vi "总磷氨氮测量数据储存.vi"   [LabVIEW 2016, in "氨氮.lvlib"]
types:
  T1 = enum16{"维护数据", "水样测试", "标样核查", "零点核查", "跨度核查", "空白测试", "平行样测试", "加标回收", "空白校准", "标样校准", "初始化（清洗）"}
  T2 = cluster{"时间标识":timestamp, "监测值":sgl, "单位":u16, "数据标识":string, "因子编码":u32, "标样参考值":sgl, "F0":sgl, "F1":sgl, "F2":sgl, "F3":sgl, "温度":sgl, "湿度":sgl, "量程标识":string}
  T3 = cluster{"运行模式":enum16{"维护模式", "常规模式", "应急模式", "质控模式"}}
  T4 = cluster{"系统时间":timestamp, "工作状态":enum16{"空闲", "水样测试", "标样核查", "零点核查", "跨度核查", "空白测试", "平行样测试", "加标回收", "空白校准", "标样校准", "初始化（清洗）"}, "测量模式":enum16{"待机", "连续模式", "周期模式", "定点模式", "受控模式", "手动模式"}, "告警代码":enum16{"无告警", "缺试剂告警", "缺水样告警", "缺蒸馏水告警", "缺标液告警", "仪表漏液告警", "标定异常告警", "超量程告警", "加热异常", "低试剂预警", "超上限告警", "超下限告警", "仪表内部其他异常", "滴定异常告警", "电极异常告警", "量程切换告警", "参数设置告警", "PH电极电位异常", "电导率电极异常", "浊度光度异常", "溶解氧电极异常", "溶解氧光强异常", "温度异常告警", "PH异常告警", "溶解氧异常告警", "电导率异常告警", "浊度异常告警", "叶绿素异常告警", "藻密度异常告警", "蓝绿藻异常告警", "ORP异常告警", "氨氮异常告警", "清洁刷异常告警", "SD卡异常告警", "蓝牙异常告警", "Wifi异常告警", "流程异常告警"}, "故障代码":enum16{"无故障", "电机故障", "温度故障", "通讯故障", "滴定故障"}, "日志代码":u16, "软件版本":u16, "F0":sgl, "F1":sgl, "F2":sgl, "F3":sgl, "T":sgl, "H":sgl, "id":u16, "flowid":u16, "量程":u16, "总磷控温温度1":sgl, "营养盐控温温度2":sgl, "ADC":sgl}
  T5 = enum16{"空闲", "水样测试", "标样核查", "零点核查", "跨度核查", "空白测试", "平行样测试", "加标回收", "空白校准", "标样校准", "初始化（清洗）"}
  T6 = cluster{"因子编码":u32, "单位":u16, "标样参考值":sgl, "水样数据时间":timestamp, "水样实测值":sgl, "水样数据标识":string, "标样数据时间":timestamp, "标样实测值":sgl, "标样数据标识":string, "空白数据时间":timestamp, "空白实测值":sgl, "空白数据标识":string, "零点核查数据时间":timestamp, "零点核查实测值":sgl, "零点核查数据标识":string, "跨度核查数据时间":timestamp, "跨度核查实测值":sgl, "跨度核查数据标识":string, "加标回收数据时间":timestamp, "加标回收实测值":sgl, "加标回收数据标识":string, "平行样数据时间":timestamp, "平行样实测值":sgl, "平行样数据标识":string}
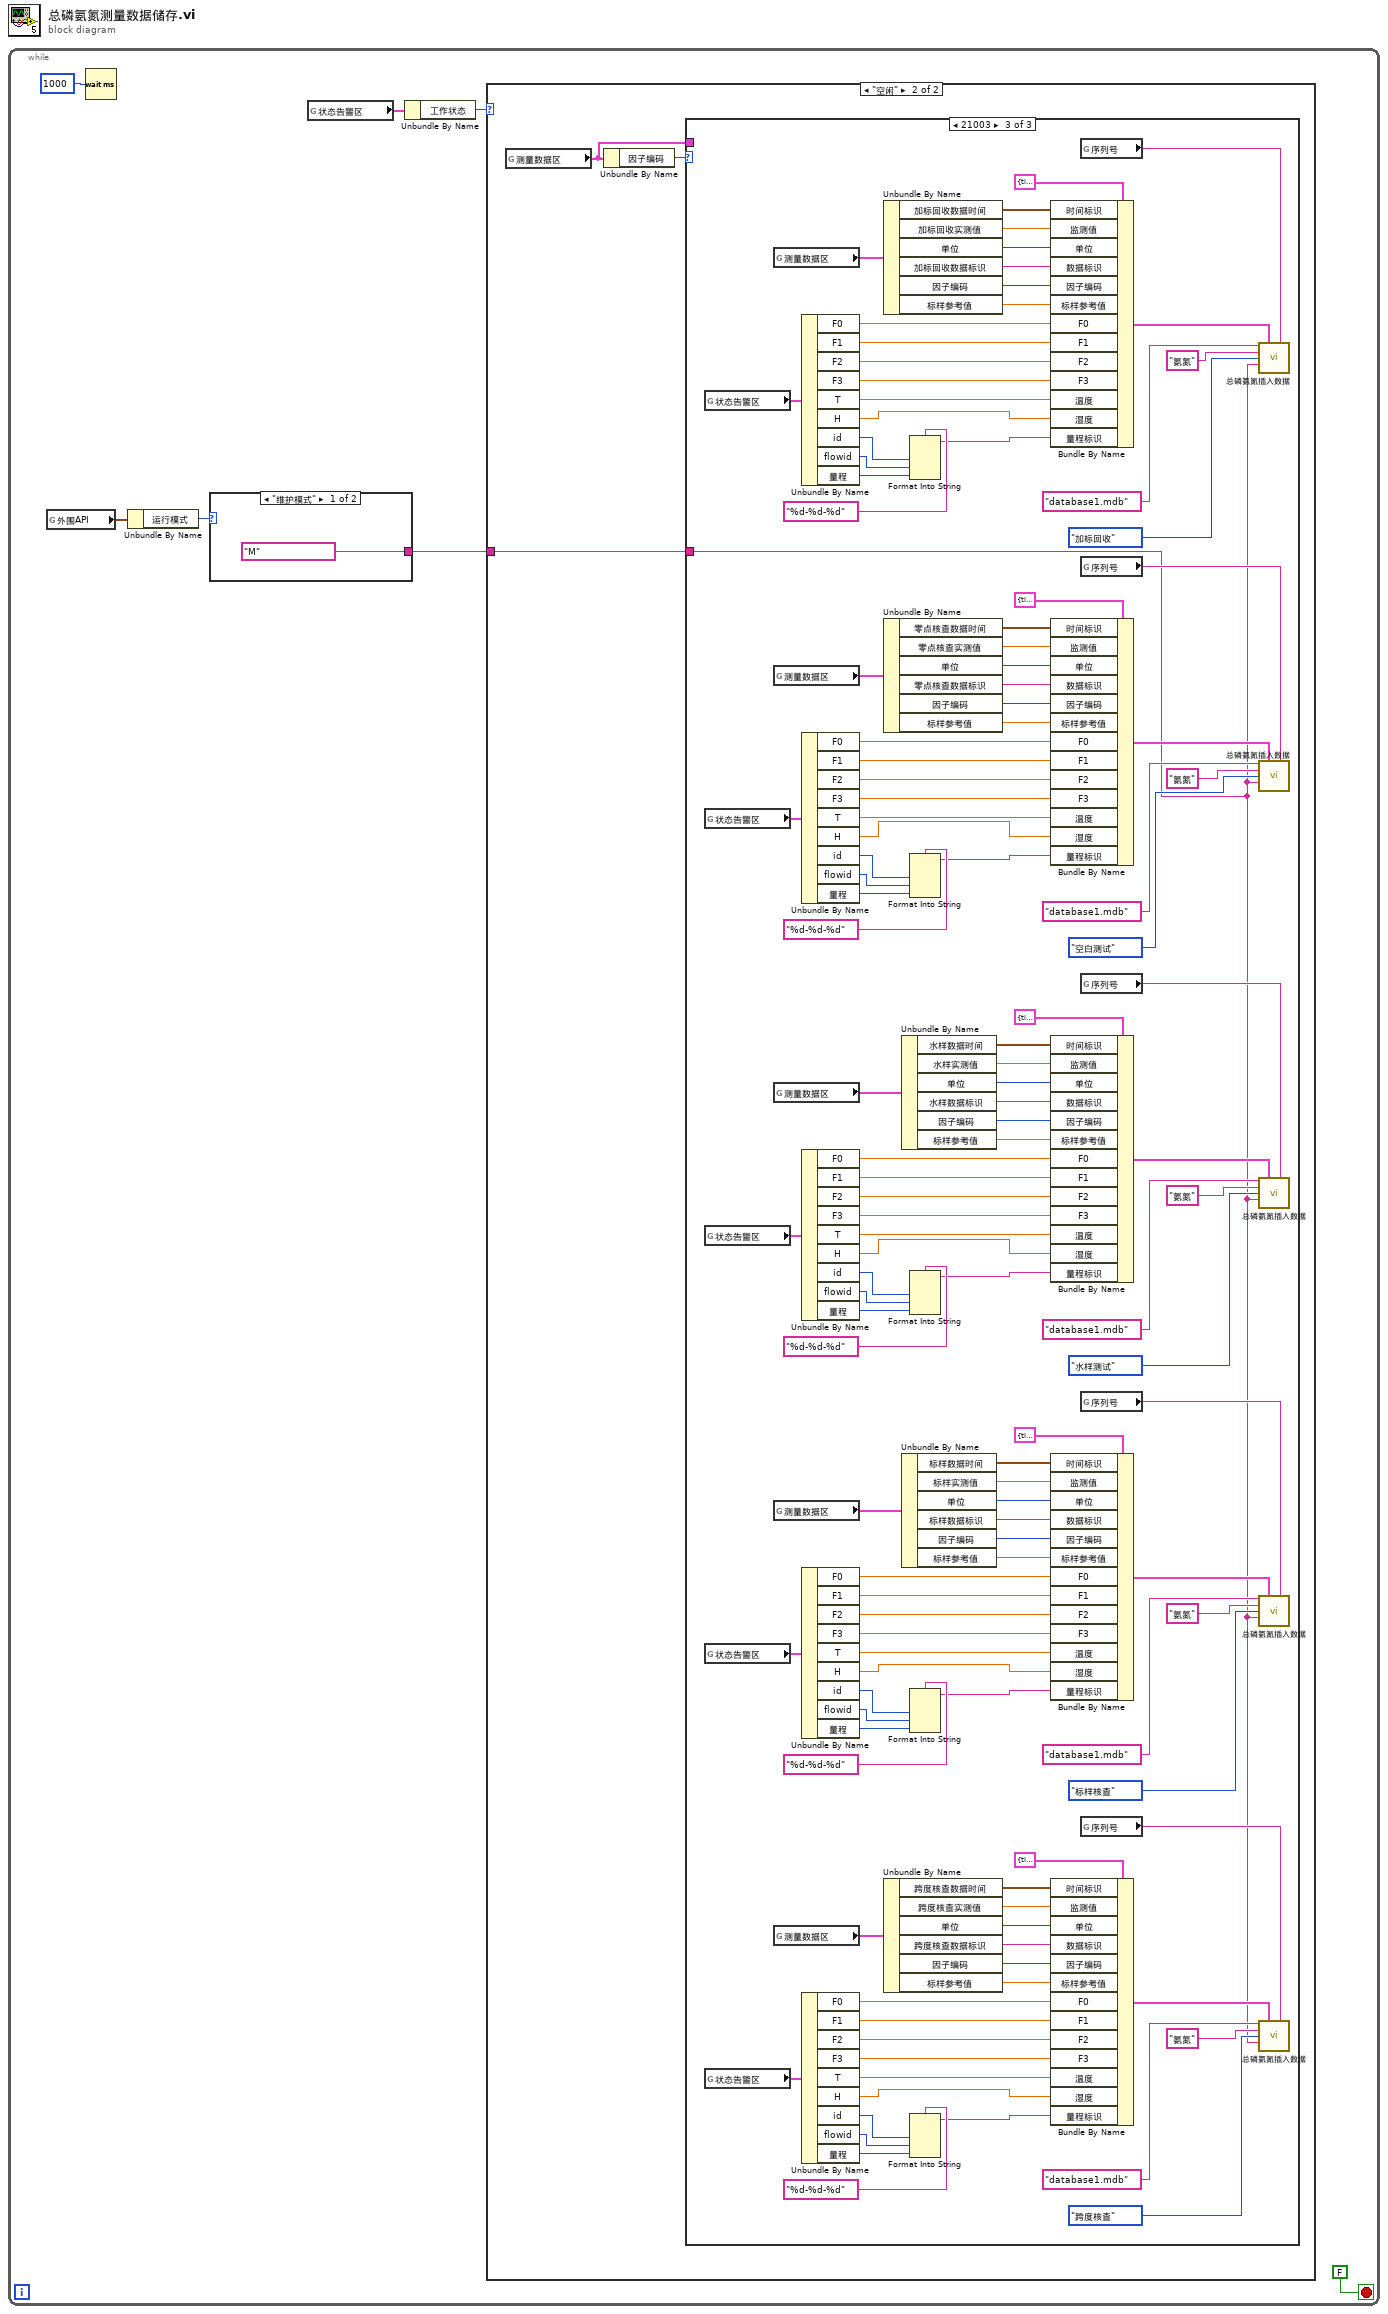
[diagram p0: block diagram]
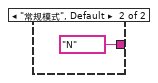
[diagram p2: hidden frame]
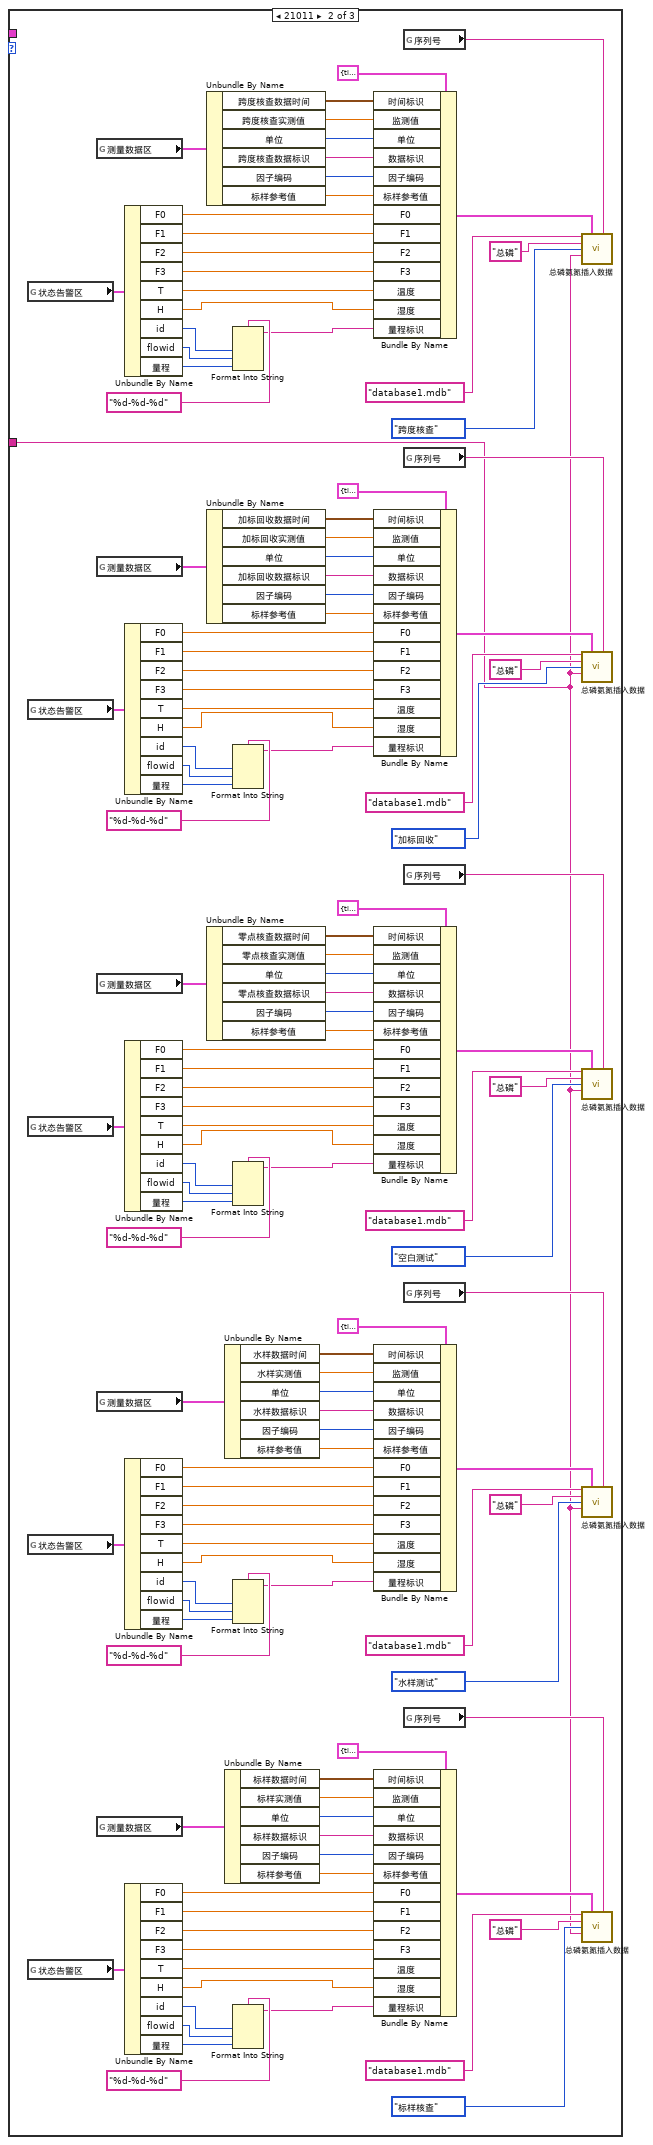
[diagram p5: hidden frame]
diagram:
  n1 = while {
    stop <- FALSE stop-if-true
    n2 = global read "VAR氨氮全局变量.vi" "外围API"() -> (w2:T3)
    n3 = Wait (ms)(milliseconds to wait=u32 1000 ("等待时间（毫秒）")) -> ()  [unwired: 1 out]
    n4 = Unbundle By Name(w2) -> ("运行模式"=w1:enum16{"维护模式", "常规模式", "应急模式", "质控模式"})
    n5 = case shown="\"维护模式\"" w1 {
      tunnel: ["M" ("数据标记表") "N" ("数据标记表")] -> w3
      frame "维护模式" {
      }
      frame "常规模式", Default {
      }
    }
    n6 = global read "VAR氨氮全局变量.vi" "状态告警区"() -> (w5:T4)
    n7 = Unbundle By Name(w5) -> ("工作状态"=w4:T5)
    n8 = case shown="\"空闲\"" w4 {
      tunnel: w3 -> [_ w10]
      frame Default {
      }
      frame "空闲" {
        n9 = global read "VAR氨氮全局变量.vi" "测量数据区"() -> (w12:T6)
        n10 = Unbundle By Name(w12) -> ("因子编码"=w11:u32)
        n11 = case shown="21003" w11 {
          tunnel: w12 -> [_ _ _]
          tunnel: w10 -> [_ w13 w139]
          frame Default {
          }
          frame 21011 {
            n12 = global read "VAR氨氮全局变量.vi" "状态告警区"() -> (w77:T4)
            n13 = global read "VAR氨氮全局变量.vi" "状态告警区"() -> (w59:T4)
            n14 = global read "VAR氨氮全局变量.vi" "状态告警区"() -> (w92:T4)
            n15 = global read "VAR氨氮全局变量.vi" "状态告警区"() -> (w131:T4)
            n16 = global read "VAR氨氮全局变量.vi" "状态告警区"() -> (w110:T4)
            n17 = global read "VAR氨氮全局变量.vi" "测量数据区"() -> (w84:T6)
            n18 = global read "VAR氨氮全局变量.vi" "测量数据区"() -> (w66:T6)
            n19 = global read "VAR氨氮全局变量.vi" "测量数据区"() -> (w85:T6)
            n20 = global read "VAR氨氮全局变量.vi" "测量数据区"() -> (w138:T6)
            n21 = global read "VAR氨氮全局变量.vi" "测量数据区"() -> (w103:T6)
            n22 = Unbundle By Name(w77) -> ("F0"=w76:sgl, "F1"=w75:sgl, "F2"=w74:sgl, "F3"=w73:sgl, "T"=w72:sgl, "H"=w71:sgl, "id"=w40:u16, "flowid"=w39:u16, "量程"=w38:u16)
            n23 = Unbundle By Name(w59) -> ("F0"=w58:sgl, "F1"=w57:sgl, "F2"=w56:sgl, "F3"=w55:sgl, "T"=w54:sgl, "H"=w53:sgl, "id"=w46:u16, "flowid"=w45:u16, "量程"=w44:u16)
            n24 = Unbundle By Name(w92) -> ("F0"=w93:sgl, "F1"=w94:sgl, "F2"=w95:sgl, "F3"=w96:sgl, "T"=w97:sgl, "H"=w98:sgl, "id"=w33:u16, "flowid"=w34:u16, "量程"=w35:u16)
            n25 = Unbundle By Name(w131) -> ("F0"=w130:sgl, "F1"=w129:sgl, "F2"=w128:sgl, "F3"=w127:sgl, "T"=w126:sgl, "H"=w125:sgl, "id"=w20:u16, "flowid"=w21:u16, "量程"=w22:u16)
            n26 = Unbundle By Name(w110) -> ("F0"=w111:sgl, "F1"=w112:sgl, "F2"=w113:sgl, "F3"=w114:sgl, "T"=w115:sgl, "H"=w116:sgl, "id"=w28:u16, "flowid"=w27:u16, "量程"=w26:u16)
            n27 = Unbundle By Name(w84) -> ("跨度核查数据时间"=w83:timestamp, "跨度核查实测值"=w82:sgl, "单位"=w81:u16, "跨度核查数据标识"=w80:string, "因子编码"=w79:u32, "标样参考值"=w78:sgl)
            n28 = Unbundle By Name(w66) -> ("加标回收数据时间"=w65:timestamp, "加标回收实测值"=w64:sgl, "单位"=w63:u16, "加标回收数据标识"=w62:string, "因子编码"=w61:u32, "标样参考值"=w60:sgl)
            n29 = Unbundle By Name(w85) -> ("零点核查数据时间"=w86:timestamp, "零点核查实测值"=w87:sgl, "单位"=w88:u16, "零点核查数据标识"=w89:string, "因子编码"=w90:u32, "标样参考值"=w91:sgl)
            n30 = Unbundle By Name(w138) -> ("水样数据时间"=w137:timestamp, "水样实测值"=w136:sgl, "单位"=w135:u16, "水样数据标识"=w134:string, "因子编码"=w133:u32, "标样参考值"=w132:sgl)
            n31 = Unbundle By Name(w103) -> ("标样数据时间"=w104:timestamp, "标样实测值"=w105:sgl, "单位"=w106:u16, "标样数据标识"=w107:string, "因子编码"=w108:u32, "标样参考值"=w109:sgl)
            n32 = Format Into String(format string="%d-%d-%d" ("格式字符串"), w40, w39, w38) -> (resulting string=w37:string)  [unwired: 2 in, 1 out]
            n33 = Format Into String(format string="%d-%d-%d" ("格式字符串"), w46, w45, w44) -> (resulting string=w43:string)  [unwired: 2 in, 1 out]
            n34 = Format Into String(format string="%d-%d-%d" ("格式字符串"), w33, w34, w35) -> (resulting string=w31:string)  [unwired: 2 in, 1 out]
            n35 = Format Into String(format string="%d-%d-%d" ("格式字符串"), w20, w21, w22) -> (resulting string=w19:string)  [unwired: 2 in, 1 out]
            n36 = Format Into String(format string="%d-%d-%d" ("格式字符串"), w28, w27, w26) -> (resulting string=w25:string)  [unwired: 2 in, 1 out]
            n37 = Bundle By Name(cluster=T2 {"时间标识"=timestamp(0 s since 1904-01-01), "监测值"=0.0, "单位"=0, "数据标识"="", "因子编码"=0, "标样参考值"=0.0, "F0"=0.0, "F1"=0.0, "F2"=0.0, "F3"=0.0, "温度"=0.0, "湿度"=0.0, "量程标识"=""} ("data"), "时间标识"=w83, "监测值"=w82, "单位"=w81, "数据标识"=w80, "因子编码"=w79, "标样参考值"=w78, "F0"=w76, "F1"=w75, "F2"=w74, "F3"=w73, "温度"=w72, "湿度"=w71, "量程标识"=w37) -> (w70:T2)
            n38 = Bundle By Name(cluster=T2 {"时间标识"=timestamp(0 s since 1904-01-01), "监测值"=0.0, "单位"=0, "数据标识"="", "因子编码"=0, "标样参考值"=0.0, "F0"=0.0, "F1"=0.0, "F2"=0.0, "F3"=0.0, "温度"=0.0, "湿度"=0.0, "量程标识"=""} ("data"), "时间标识"=w65, "监测值"=w64, "单位"=w63, "数据标识"=w62, "因子编码"=w61, "标样参考值"=w60, "F0"=w58, "F1"=w57, "F2"=w56, "F3"=w55, "温度"=w54, "湿度"=w53, "量程标识"=w43) -> (w52:T2)
            n39 = Bundle By Name(cluster=T2 {"时间标识"=timestamp(0 s since 1904-01-01), "监测值"=0.0, "单位"=0, "数据标识"="", "因子编码"=0, "标样参考值"=0.0, "F0"=0.0, "F1"=0.0, "F2"=0.0, "F3"=0.0, "温度"=0.0, "湿度"=0.0, "量程标识"=""} ("data"), "时间标识"=w86, "监测值"=w87, "单位"=w88, "数据标识"=w89, "因子编码"=w90, "标样参考值"=w91, "F0"=w93, "F1"=w94, "F2"=w95, "F3"=w96, "温度"=w97, "湿度"=w98, "量程标识"=w31) -> (w99:T2)
            n40 = Bundle By Name(cluster=T2 {"时间标识"=timestamp(0 s since 1904-01-01), "监测值"=0.0, "单位"=0, "数据标识"="", "因子编码"=0, "标样参考值"=0.0, "F0"=0.0, "F1"=0.0, "F2"=0.0, "F3"=0.0, "温度"=0.0, "湿度"=0.0, "量程标识"=""} ("data"), "时间标识"=w137, "监测值"=w136, "单位"=w135, "数据标识"=w134, "因子编码"=w133, "标样参考值"=w132, "F0"=w130, "F1"=w129, "F2"=w128, "F3"=w127, "温度"=w126, "湿度"=w125, "量程标识"=w19) -> (w124:T2)
            n41 = Bundle By Name(cluster=T2 {"时间标识"=timestamp(0 s since 1904-01-01), "监测值"=0.0, "单位"=0, "数据标识"="", "因子编码"=0, "标样参考值"=0.0, "F0"=0.0, "F1"=0.0, "F2"=0.0, "F3"=0.0, "温度"=0.0, "湿度"=0.0, "量程标识"=""} ("data"), "时间标识"=w104, "监测值"=w105, "单位"=w106, "数据标识"=w107, "因子编码"=w108, "标样参考值"=w109, "F0"=w111, "F1"=w112, "F2"=w113, "F3"=w114, "温度"=w115, "湿度"=w116, "量程标识"=w25) -> (w117:T2)
            n42 = global read "VAR氨氮全局变量.vi" "序列号"() -> (w15:string)
            n43 = global read "VAR氨氮全局变量.vi" "序列号"() -> (w14:string)
            n44 = global read "VAR氨氮全局变量.vi" "序列号"() -> (w16:string)
            n45 = global read "VAR氨氮全局变量.vi" "序列号"() -> (w18:string)
            n46 = global read "VAR氨氮全局变量.vi" "序列号"() -> (w17:string)
            n47 = call "总磷氨氮插入数据.vi"("database"="database1.mdb", "data"=w70, "SN"=w15, "table"="总磷", "测量模式"=T1."跨度核查", "数据标记表"=w13) -> ()  [unwired: 9 in, 1 out]
            n48 = call "总磷氨氮插入数据.vi"("database"="database1.mdb", "data"=w52, "SN"=w14, "table"="总磷", "测量模式"=T1."加标回收", "数据标记表"=w13) -> ()  [unwired: 9 in, 1 out]
            n49 = call "总磷氨氮插入数据.vi"("database"="database1.mdb", "data"=w99, "SN"=w16, "table"="总磷", "测量模式"=T1."空白测试", "数据标记表"=w13) -> ()  [unwired: 9 in, 1 out]
            n50 = call "总磷氨氮插入数据.vi"("database"="database1.mdb", "data"=w124, "SN"=w18, "table"="总磷", "测量模式"=T1."水样测试", "数据标记表"=w13) -> ()  [unwired: 9 in, 1 out]
            n51 = call "总磷氨氮插入数据.vi"("database"="database1.mdb", "data"=w117, "SN"=w17, "table"="总磷", "测量模式"=T1."标样核查", "数据标记表"=w13) -> ()  [unwired: 9 in, 1 out]
          }
          frame 21003 {
            n52 = global read "VAR氨氮全局变量.vi" "状态告警区"() -> (w185:T4)
            n53 = global read "VAR氨氮全局变量.vi" "状态告警区"() -> (w218:T4)
            n54 = global read "VAR氨氮全局变量.vi" "状态告警区"() -> (w257:T4)
            n55 = global read "VAR氨氮全局变量.vi" "状态告警区"() -> (w236:T4)
            n56 = global read "VAR氨氮全局变量.vi" "状态告警区"() -> (w203:T4)
            n57 = global read "VAR氨氮全局变量.vi" "测量数据区"() -> (w192:T6)
            n58 = global read "VAR氨氮全局变量.vi" "测量数据区"() -> (w211:T6)
            n59 = global read "VAR氨氮全局变量.vi" "测量数据区"() -> (w264:T6)
            n60 = global read "VAR氨氮全局变量.vi" "测量数据区"() -> (w229:T6)
            n61 = global read "VAR氨氮全局变量.vi" "测量数据区"() -> (w210:T6)
            n62 = Unbundle By Name(w185) -> ("F0"=w184:sgl, "F1"=w183:sgl, "F2"=w182:sgl, "F3"=w181:sgl, "T"=w180:sgl, "H"=w179:sgl, "id"=w160:u16, "flowid"=w159:u16, "量程"=w158:u16)
            n63 = Unbundle By Name(w218) -> ("F0"=w219:sgl, "F1"=w220:sgl, "F2"=w221:sgl, "F3"=w222:sgl, "T"=w223:sgl, "H"=w224:sgl, "id"=w148:u16, "flowid"=w147:u16, "量程"=w146:u16)
            n64 = Unbundle By Name(w257) -> ("F0"=w256:sgl, "F1"=w255:sgl, "F2"=w254:sgl, "F3"=w253:sgl, "T"=w252:sgl, "H"=w251:sgl, "id"=w173:u16, "flowid"=w172:u16, "量程"=w171:u16)
            n65 = Unbundle By Name(w236) -> ("F0"=w237:sgl, "F1"=w238:sgl, "F2"=w239:sgl, "F3"=w240:sgl, "T"=w241:sgl, "H"=w242:sgl, "id"=w166:u16, "flowid"=w165:u16, "量程"=w164:u16)
            n66 = Unbundle By Name(w203) -> ("F0"=w202:sgl, "F1"=w201:sgl, "F2"=w200:sgl, "F3"=w199:sgl, "T"=w198:sgl, "H"=w197:sgl, "id"=w154:u16, "flowid"=w153:u16, "量程"=w152:u16)
            n67 = Unbundle By Name(w192) -> ("加标回收数据时间"=w191:timestamp, "加标回收实测值"=w190:sgl, "单位"=w189:u16, "加标回收数据标识"=w188:string, "因子编码"=w187:u32, "标样参考值"=w186:sgl)
            n68 = Unbundle By Name(w211) -> ("零点核查数据时间"=w212:timestamp, "零点核查实测值"=w213:sgl, "单位"=w214:u16, "零点核查数据标识"=w215:string, "因子编码"=w216:u32, "标样参考值"=w217:sgl)
            n69 = Unbundle By Name(w210) -> ("跨度核查数据时间"=w209:timestamp, "跨度核查实测值"=w208:sgl, "单位"=w207:u16, "跨度核查数据标识"=w206:string, "因子编码"=w205:u32, "标样参考值"=w204:sgl)
            n70 = Unbundle By Name(w264) -> ("水样数据时间"=w263:timestamp, "水样实测值"=w262:sgl, "单位"=w261:u16, "水样数据标识"=w260:string, "因子编码"=w259:u32, "标样参考值"=w258:sgl)
            n71 = Unbundle By Name(w229) -> ("标样数据时间"=w230:timestamp, "标样实测值"=w231:sgl, "单位"=w232:u16, "标样数据标识"=w233:string, "因子编码"=w234:u32, "标样参考值"=w235:sgl)
            n72 = Format Into String(format string="%d-%d-%d" ("格式字符串"), w160, w159, w158) -> (resulting string=w157:string)  [unwired: 2 in, 1 out]
            n73 = Format Into String(format string="%d-%d-%d" ("格式字符串"), w148, w147, w146) -> (resulting string=w145:string)  [unwired: 2 in, 1 out]
            n74 = Format Into String(format string="%d-%d-%d" ("格式字符串"), w173, w172, w171) -> (resulting string=w169:string)  [unwired: 2 in, 1 out]
            n75 = Format Into String(format string="%d-%d-%d" ("格式字符串"), w166, w165, w164) -> (resulting string=w163:string)  [unwired: 2 in, 1 out]
            n76 = Format Into String(format string="%d-%d-%d" ("格式字符串"), w154, w153, w152) -> (resulting string=w151:string)  [unwired: 2 in, 1 out]
            n77 = Bundle By Name(cluster=T2 {"时间标识"=timestamp(0 s since 1904-01-01), "监测值"=0.0, "单位"=0, "数据标识"="", "因子编码"=0, "标样参考值"=0.0, "F0"=0.0, "F1"=0.0, "F2"=0.0, "F3"=0.0, "温度"=0.0, "湿度"=0.0, "量程标识"=""} ("data"), "时间标识"=w191, "监测值"=w190, "单位"=w189, "数据标识"=w188, "因子编码"=w187, "标样参考值"=w186, "F0"=w184, "F1"=w183, "F2"=w182, "F3"=w181, "温度"=w180, "湿度"=w179, "量程标识"=w157) -> (w178:T2)
            n78 = Bundle By Name(cluster=T2 {"时间标识"=timestamp(0 s since 1904-01-01), "监测值"=0.0, "单位"=0, "数据标识"="", "因子编码"=0, "标样参考值"=0.0, "F0"=0.0, "F1"=0.0, "F2"=0.0, "F3"=0.0, "温度"=0.0, "湿度"=0.0, "量程标识"=""} ("data"), "时间标识"=w212, "监测值"=w213, "单位"=w214, "数据标识"=w215, "因子编码"=w216, "标样参考值"=w217, "F0"=w219, "F1"=w220, "F2"=w221, "F3"=w222, "温度"=w223, "湿度"=w224, "量程标识"=w145) -> (w225:T2)
            n79 = Bundle By Name(cluster=T2 {"时间标识"=timestamp(0 s since 1904-01-01), "监测值"=0.0, "单位"=0, "数据标识"="", "因子编码"=0, "标样参考值"=0.0, "F0"=0.0, "F1"=0.0, "F2"=0.0, "F3"=0.0, "温度"=0.0, "湿度"=0.0, "量程标识"=""} ("data"), "时间标识"=w263, "监测值"=w262, "单位"=w261, "数据标识"=w260, "因子编码"=w259, "标样参考值"=w258, "F0"=w256, "F1"=w255, "F2"=w254, "F3"=w253, "温度"=w252, "湿度"=w251, "量程标识"=w169) -> (w250:T2)
            n80 = Bundle By Name(cluster=T2 {"时间标识"=timestamp(0 s since 1904-01-01), "监测值"=0.0, "单位"=0, "数据标识"="", "因子编码"=0, "标样参考值"=0.0, "F0"=0.0, "F1"=0.0, "F2"=0.0, "F3"=0.0, "温度"=0.0, "湿度"=0.0, "量程标识"=""} ("data"), "时间标识"=w230, "监测值"=w231, "单位"=w232, "数据标识"=w233, "因子编码"=w234, "标样参考值"=w235, "F0"=w237, "F1"=w238, "F2"=w239, "F3"=w240, "温度"=w241, "湿度"=w242, "量程标识"=w163) -> (w243:T2)
            n81 = Bundle By Name(cluster=T2 {"时间标识"=timestamp(0 s since 1904-01-01), "监测值"=0.0, "单位"=0, "数据标识"="", "因子编码"=0, "标样参考值"=0.0, "F0"=0.0, "F1"=0.0, "F2"=0.0, "F3"=0.0, "温度"=0.0, "湿度"=0.0, "量程标识"=""} ("data"), "时间标识"=w209, "监测值"=w208, "单位"=w207, "数据标识"=w206, "因子编码"=w205, "标样参考值"=w204, "F0"=w202, "F1"=w201, "F2"=w200, "F3"=w199, "温度"=w198, "湿度"=w197, "量程标识"=w151) -> (w196:T2)
            n82 = global read "VAR氨氮全局变量.vi" "序列号"() -> (w140:string)
            n83 = global read "VAR氨氮全局变量.vi" "序列号"() -> (w142:string)
            n84 = global read "VAR氨氮全局变量.vi" "序列号"() -> (w144:string)
            n85 = global read "VAR氨氮全局变量.vi" "序列号"() -> (w143:string)
            n86 = global read "VAR氨氮全局变量.vi" "序列号"() -> (w141:string)
            n87 = call "总磷氨氮插入数据.vi"("database"="database1.mdb", "data"=w178, "SN"=w140, "table"="氨氮", "测量模式"=T1."加标回收", "数据标记表"=w139) -> ()  [unwired: 9 in, 1 out]
            n88 = call "总磷氨氮插入数据.vi"("database"="database1.mdb", "data"=w225, "SN"=w142, "table"="氨氮", "测量模式"=T1."空白测试", "数据标记表"=w139) -> ()  [unwired: 9 in, 1 out]
            n89 = call "总磷氨氮插入数据.vi"("database"="database1.mdb", "data"=w250, "SN"=w144, "table"="氨氮", "测量模式"=T1."水样测试", "数据标记表"=w139) -> ()  [unwired: 9 in, 1 out]
            n90 = call "总磷氨氮插入数据.vi"("database"="database1.mdb", "data"=w243, "SN"=w143, "table"="氨氮", "测量模式"=T1."标样核查", "数据标记表"=w139) -> ()  [unwired: 9 in, 1 out]
            n91 = call "总磷氨氮插入数据.vi"("database"="database1.mdb", "data"=w196, "SN"=w141, "table"="氨氮", "测量模式"=T1."跨度核查", "数据标记表"=w139) -> ()  [unwired: 9 in, 1 out]
          }
        }
      }
    }
  }
